vi "Update Force Calibration Results.vi"(7 "new results?":bool, 8 "error in (no error)":errorcluster, 9 "fs cal results":dbl[][](array[numeric]), 10 "main gui queue":refnum<queue>, 11 "gui notifier":refnum<notifier>) -> (0 "error out":errorcluster)   [LabVIEW 2020]
uses:
  GUI/Main GUI Loop/Handler.ctl
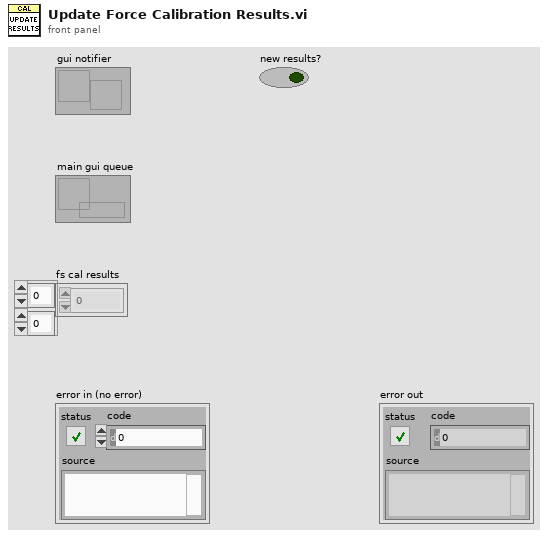
[diagram p1: front panel]
types:
  T1 = typedef "Handler.ctl" = cluster{"bool ref":refnum<vi>, "error":errorcluster, "msg":string, "status":string, "switch status":bool, "force cal":dbl[][], "force cal results":dbl[][]}
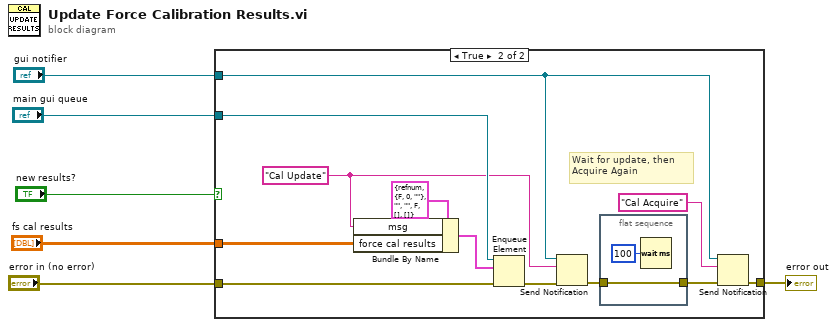
[diagram p0: block diagram]
diagram:
  n1 = case shown="True" "new results?" {
    tunnel: "error in (no error)" -> [w7 w19]
    tunnel: "main gui queue" -> [_ w18]
    tunnel: "fs cal results" -> [_ w15]
    tunnel: "gui notifier" -> [_ w9]
    tunnel: [w7 w10] -> w5
    frame False {
      # "Do nothing if no new results"
    }
    frame True {
      w13 = "Cal Update" ("msg")
      # "Wait for update, then Acquire Again"
      n2 = Bundle By Name(cluster=T1 {"bool ref"=refnum, "error"={"status"=FALSE, "code"=0, "source"=""}, "msg"="", "status"="", "switch status"=FALSE, "force cal"=[], "force cal results"=[]} ("element"), "msg"=w13, "force cal results"=w15) -> (w16:T1)
      n3 = Enqueue Element(queue=w18, element=w16, error in (no error)=w19) -> (error out=w14:errorcluster)  [unwired: 1 in, 2 out]
      n4 = Send Notification(notification=w13, notifier=w9, error in (no error)=w14) -> (error out=w12:errorcluster)  [unwired: 1 out]
      n5 = flat-sequence {
        tunnel: w12 -> [w21]
        tunnel: [w21] -> w11
        frame #0 {
          n6 = Wait (ms)(milliseconds to wait=u32 100) -> ()  [unwired: 1 out]
        }
      }
      n7 = Send Notification(notification="Cal Acquire", notifier=w9, error in (no error)=w11) -> (error out=w10:errorcluster)  [unwired: 1 out]
    }
  }
  "error out" <- w5
